vi "GetConsoleError.vi"(8 "error in (no error)":errorcluster, 11 "String in":string) -> (3 "String out":string)   [LabVIEW 2012]
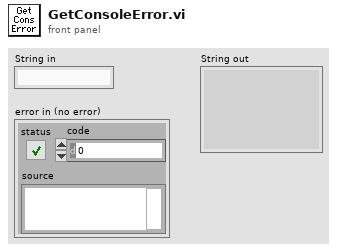
[diagram p1: front panel]
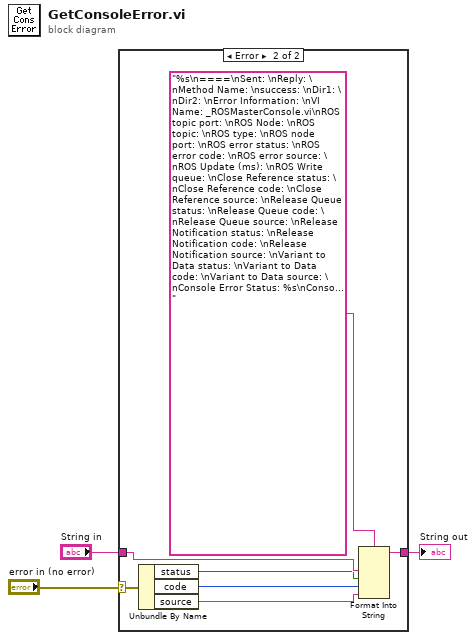
[diagram p0: block diagram]
diagram:
  n1 = case shown="Error" "error in (no error)" {
    selector: "error in (no error)" -> [_ w11]
    tunnel: "String in" -> [w4 w7]
    tunnel: [w4 w5] -> w3
    frame No Error {
    }
    frame Error {
      n2 = Unbundle By Name(w11) -> ("status"=w6:bool, "code"=w10:i32, "source"=w9:string)
      n3 = Format Into String(format string="%s\n====\nSent: \nReply: \nMethod Name: \nsuccess: \nDir1: \nDir2: \nError Information: \nVI Name: _ROSMasterConsole.vi\nROS topic port: \nROS Node: \nROS topic: \nROS type: \nROS node port: \nROS error status: \nROS error code: \nROS error source: \nROS Update (ms): \nROS Write queue: \nClose Reference status: \nClose Reference code: \nClose Reference source: \nRelease Queue status: \nRelease Queue code: \nRelease Queue source: \nRelease Notification status: \nRelease Notification code: \nRelease Notification source: \nVariant to Data status: \nVariant to Data code: \nVariant to Data source: \nConsole Error Status: %s\nConsole Error Code: %d\nConsole Error Source: %s\nTimestamp: \n====", w7, w6, w10, w9) -> (resulting string=w5:string)  [unwired: 2 in, 1 out]
    }
  }
  "String out" <- w3
